vi "Get Distance.vi"(8 "error in (no error)":errorcluster, 11 "DriveMotors in":refnum<class "DriveMotors.lvclass">) -> (0 "error out":errorcluster, 2 "Distance":dbl, 3 "DriveMotors out":refnum<class "DriveMotors.lvclass">)   [LabVIEW 2013, in "DriveMotors.lvclass"]
uses:
  DriveMotors.lvclass
  DriveMotors.lvclass/DriveMotors.ctl
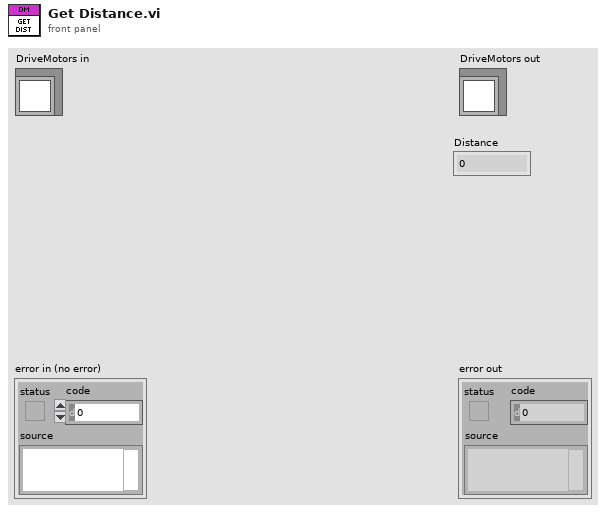
[diagram p1: front panel]
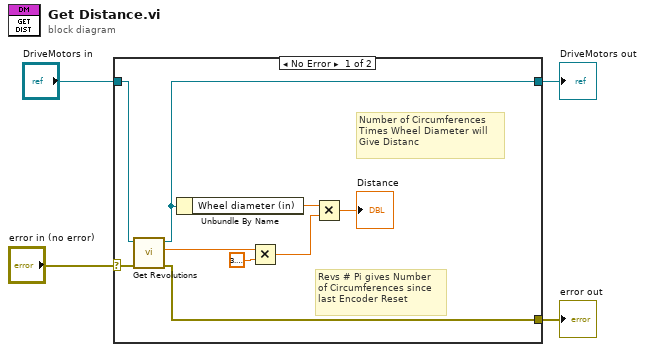
[diagram p0: block diagram]
diagram:
  n1 = case shown="No Error" "error in (no error)" {
    selector: "error in (no error)" -> [w12 w15]
    tunnel: [w5 w15] -> w3
    tunnel: [w11 w14] -> w1
    tunnel: "DriveMotors in" -> [w13 w14]
    frame No Error {
      # "Number of Circumferences\nTimes Wheel Diameter will\nGive Distanc"
      # "Revs # Pi gives Number\nof Circumferences since\nlast Encoder Reset"
      n2 = call-dynamic "Get Revolutions.vi"("error in (no error)"=w12, "DriveMotors in"=w13) -> ("error out"=w5:errorcluster, "Revolutions"=w9:dbl, "DriveMotors out"=w11:refnum<class "DriveMotors.lvclass">)  [unwired: 7 in]
      n3 = Unbundle By Name(w11) -> ("Wheel diameter (in)"=w7:dbl)
      n4 = Multiply(x=w9, y=3.141592653589793) -> (x*y=w8:dbl)
      n5 = Multiply(x=w7, y=w8) -> (x*y=→"Distance":dbl)
    }
    frame Error {
    }
  }
  "error out" <- w3
  "DriveMotors out" <- w1
